vi "User32.SendMessageA_str.vi"(0 "HWnd":i32, 5 "Msg":i32, 7 "WParam":i32, 9 "LParam":string, 11 "ErrorIn":errorcluster) -> (10 "StrOut":string, 15 "ErrorOut":errorcluster)   [LabVIEW 2021]
uses:
  user32.dll
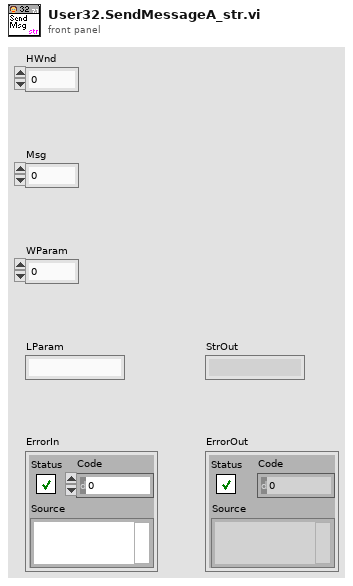
[diagram p1: front panel]
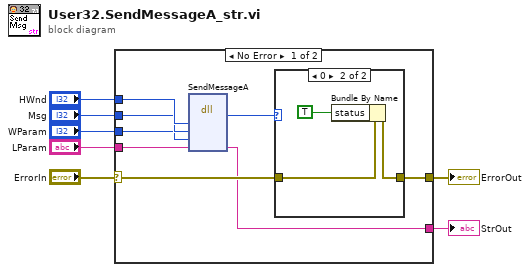
[diagram p0: block diagram]
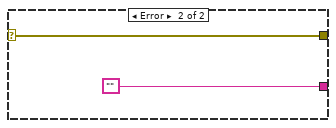
[diagram p3: hidden frame]
diagram:
  n1 = case shown="No Error" "ErrorIn" {
    selector: "ErrorIn" -> [w15 w21]
    tunnel: "HWnd" -> [w13 _]
    tunnel: "Msg" -> [w12 _]
    tunnel: "WParam" -> [w11 _]
    tunnel: [w14 w21] -> w6
    tunnel: "LParam" -> [w9 _]
    tunnel: [w8 ""] -> w1
    frame No Error {
      n2 = dll-call lib="user32.dll" fn="SendMessageA"("hWnd"=w13, "Msg"=w12, "wParam"=w11, "lParam"=w9) -> (w10:i32, "lParam"=w8:string)  [unwired: 6 in, 2 out]
      n3 = case shown="0" w10 {
        tunnel: w15 -> [w16 w19]
        tunnel: [w16 w18] -> w14
        frame Default {
        }
        frame 0 {
          n4 = Bundle By Name(cluster=w19, "status"=TRUE) -> (w18:errorcluster)
        }
      }
    }
    frame Error {
    }
  }
  "ErrorOut" <- w6
  "StrOut" <- w1
